vi "Setup UI.vi"(8 "error in (no error)":errorcluster, 11 "Operator UI in":refnum<class "Server UI.lvclass">) -> (0 "error out":errorcluster, 3 "Operator UI out":refnum<class "Server UI.lvclass">)   [LabVIEW 2026, in "Server UI.lvlib" / "Server UI.lvclass"]
uses:
  Server UI.lvclass
  C:/Users/E2013170/Documents/GitHub/Measurement-Utility-Reference/source/framework/User Interface/UI.lvclass
  <vilib>/Utility/miscctls.llb/LVRowAndColumnUnsignedTypeDef.ctl
  Server UI.lvclass/Server UI.ctl
  framework/User Interface/UI.lvclass/UI.ctl
  Write Connection Showing.vi
  Read Start Server.vi
  Read Connected Clients.vi
  framework/Msmt UI/Measurement UI.lvclass
  framework/User Interface/UI.lvclass
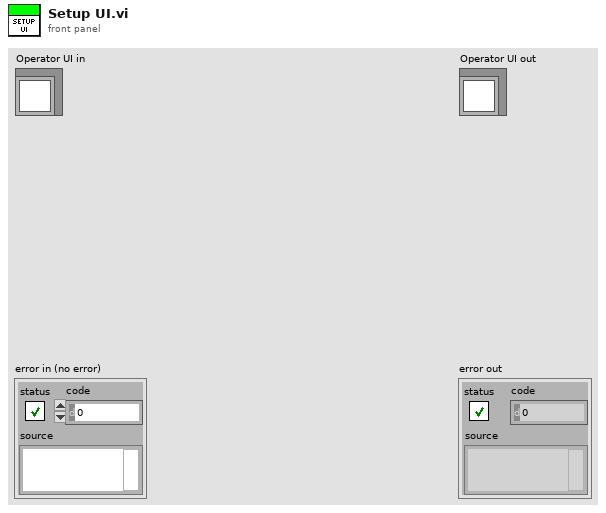
[diagram p1: front panel]
types:
  T1 = typedef "LVRowAndColumnUnsignedTypeDef.ctl" = cluster{"Row":u32, "Column":u32}
  T2 = typedef "LVRectTypeDef.ctl" = cluster{"Left":i16, "Top":i16, "Right":i16, "Bottom":i16}
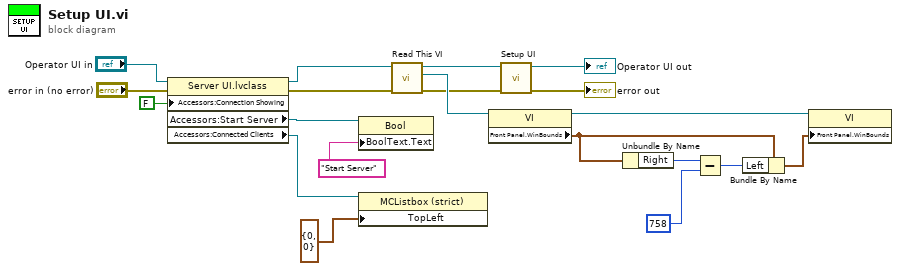
[diagram p0: block diagram]
diagram:
  n1 = property class="Server UI.lvclass"(reference="Operator UI in", error in="error in (no error)", "Accessors:Connection Showing"=FALSE ("Connection Showing")) -> (reference out=w11:refnum<class "Server UI.lvclass">, error out=w8:errorcluster, "Accessors:Start Server"=w4:refnum<vi>, "Accessors:Connected Clients"=w2:refnum<vi>)
  n2 = property class="Bool"(reference=w4, "BoolText.Text"="Start Server" ("Boolean Text.Text")) -> ()  [unwired: 1 in, 2 out]
  n3 = property class="MCListbox (strict)"(reference=w2, "TopLeft"=T1 {"Row"=0, "Column"=0} ("Top Left Visible Cell")) -> ()  [unwired: 1 in, 2 out]
  n4 = call "Read This VI.vi"("error in (no error)"=w8, "UI in"=w11) -> ("error out"=w6:errorcluster, "This VI"=w10:refnum<vi>, "UI out"=w9:refnum<class "Server UI.lvclass">)  [unwired: 7 in]
  n5 = property class="VI"(reference=w10) -> (reference out=w5:refnum<vi>, "Front Panel.WinBounds"=w18:T2)  [unwired: 1 in, 1 out]
  n6 = call-parent "Setup UI.vi"("error in (no error)"=w6, "Operator UI in"=w9) -> ("error out"=→"error out":errorcluster, "Operator UI out"=→"Operator UI out":refnum<class "Server UI.lvclass">)  [unwired: 8 in]
  n7 = Unbundle By Name(w18) -> ("Right"=w15:i16)
  n8 = Subtract(x=w15, y=i16 758) -> (x-y=w16:i16)
  n9 = Bundle By Name(cluster=w18, "Left"=w16) -> (w17:T2)
  n10 = property class="VI"(reference=w5, "Front Panel.WinBounds"=w17) -> ()  [unwired: 1 in, 2 out]
